vi "Write Graph Plot Names (UTF-8 String).vi"(8 "error in":errorcluster, 10 "Plot Names":refnum<class "UTF-8 String.lvclass">[](array[class]), 11 "Control Ref":refnum<vi>) -> (0 "error out":errorcluster)   [LabVIEW 2020, in "G-Unicode.lvlib"]
doc: "Write and display unicode text in the graph plot names of a graph control. <b>Value</b> should contain an element per plot name.\n\n<b>NOTE:</b> Requires copying unicode text from a LabVIEW string displaying unicode, and pasting it over the plot name text to activate unicode display.\n\n<b>WARNING:</b> Unicode setting of plot name doesn't persist when VI saved."
uses:
  G-Unicode.lvlib
  Types/UTF-8 String/UTF-8 String.lvclass
  Types/UTF-8 String/UTF-8 String.lvclass/UTF-8 String.ctl
  5206cb6b-04fb-41f5-a37e-29c14f142303.vi
  Private/Conversion/Text as Encoded String.vi
  Private/Conversion/Polymorphic VIs/Text as Encoded String (UTF-8 String).vi
  Private/Conversion/Encoded UTF-8 String to Encoded UTF-16LE String.vi
  Types/UTF-8 String/Read Encoded UTF-8 String.vi
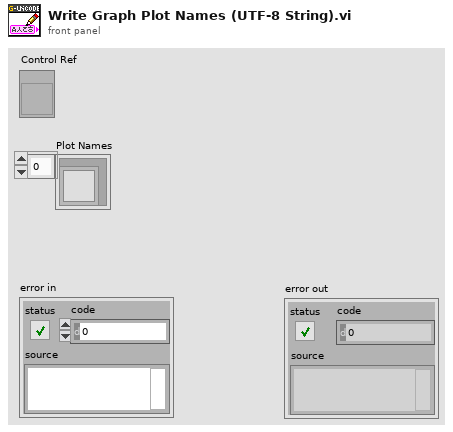
[diagram p1: front panel]
types:
  T1 = typedef "G-Unicode.lvlib/Encoded UTF-16LE String.ctl" = string
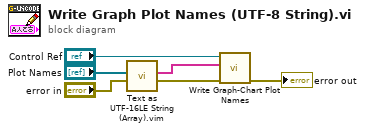
[diagram p0: block diagram]
diagram:
  n1 = call "Text as UTF-16LE String (Array).vim"("error in"="error in", "Text"="Plot Names") -> ("error out"=w1:errorcluster, "Encoded String"=w4:T1[])  [unwired: 8 in]
  n2 = call "Write Graph-Chart Plot Names.vi"("error in"=w1, "Value"=w4, "Graph / Chart Reference in"="Control Ref") -> ("error out"=→"error out":errorcluster)  [unwired: 7 in, 1 out]
